vi "FlatToRichni_measurementlink_pinmap_v1_QueryResourceAccessInformationRequest.vi"(5 "OutputClusterType":T1, 11 "InputCluster":T2) -> (3 "OutputCluster":T1)   [LabVIEW 2021, in "ni.measurementlink.pinmap.v1.api.lvlib"]
uses:
  ni_measurementlink_pinmap_v1_QueryResourceAccessInformationRequest_Flat.ctl
  ni_measurementlink_pinmap_v1_QueryResourceAccessInformationRequest.ctl
  ni.measurementlink.pinmap.v1.api.lvlib
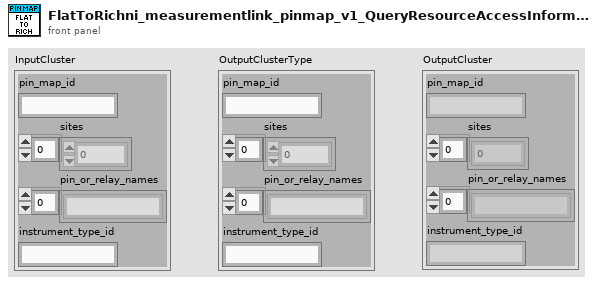
[diagram p1: front panel]
types:
  T1 = typedef "ni.measurementlink.pinmap.v1.api.lvlib/ni_measurementlink_pinmap_v1_QueryResourceAccessInformationRequest.ctl" = cluster{"pin_map_id":string, "sites":i32[], "pin_or_relay_names":string[], "instrument_type_id":string}
  T2 = typedef "ni.measurementlink.pinmap.v1.api.lvlib/ni_measurementlink_pinmap_v1_QueryResourceAccessInformationRequest_Flat.ctl" = cluster{"pin_map_id":string, "sites":i32[], "pin_or_relay_names":string[], "instrument_type_id":string}
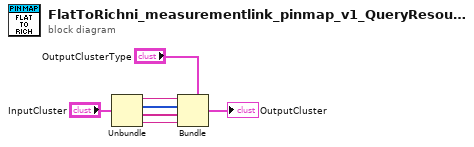
[diagram p0: block diagram]
diagram:
  n1 = Unbundle "Unbundle"("InputCluster") -> ("pin_map_id"=w4:string, "sites"=w3:i32[], "pin_or_relay_names"=w2:string[], "instrument_type_id"=w1:string)
  n2 = Bundle "Bundle"(cluster="OutputClusterType", "pin_map_id"=w4, "sites"=w3, "pin_or_relay_names"=w2, "instrument_type_id"=w1) -> (→"OutputCluster":T1)
